vi "KAL Daten loggen.vi"(4 "Aktionen MFC loggen":T1, 6 "TimeOUT":bool, 7 "Komponente":string, 8 "Kalibrieren Erfolgreich":bool, 9 "Prüfgaskonzentration":sgl, 10 "Kalibrierwert":sgl, 11 "Rohwert":sgl) -> (3 "Pfad+Name":path)   [LabVIEW 2020, in "Auto Kalibrieren.lvlib"]
uses:
  Auto Kalibrieren.lvlib
  KAL Daten loggen Aktionen.ctl
  Allgemein/allgemeine Sub-VIs.lvlib
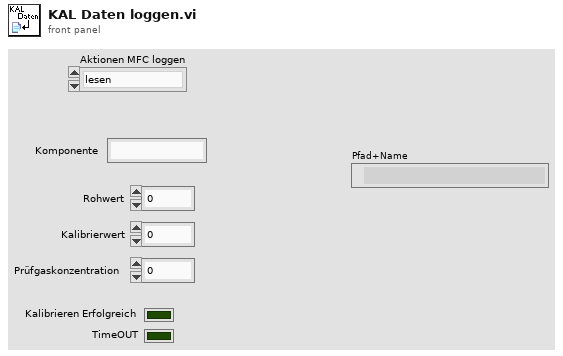
[diagram p1: front panel]
types:
  T1 = typedef "Auto Kalibrieren.lvlib/KAL Daten loggen Aktionen.ctl" = enum16{"lesen", "initialisieren", "loggen"}
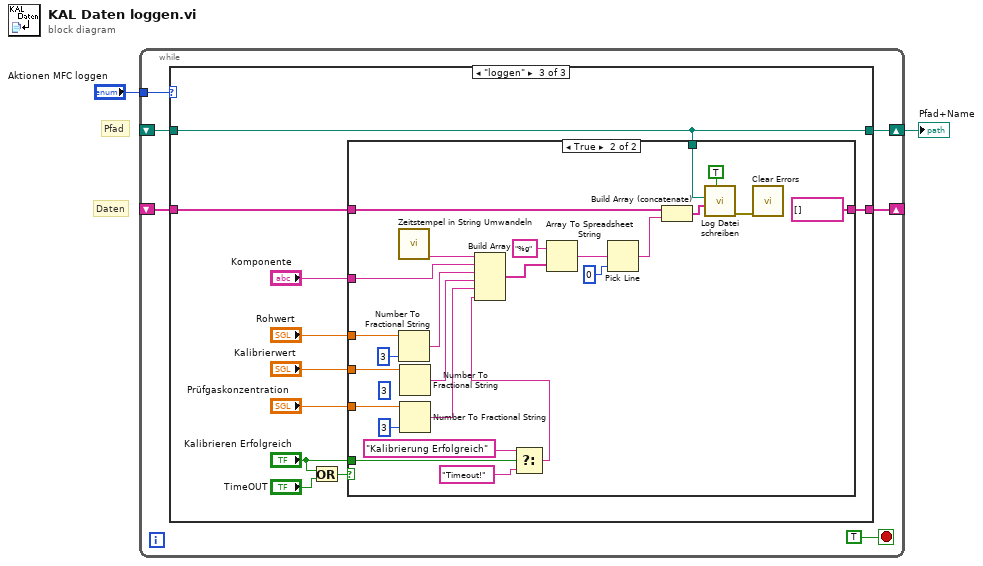
[diagram p0: block diagram]
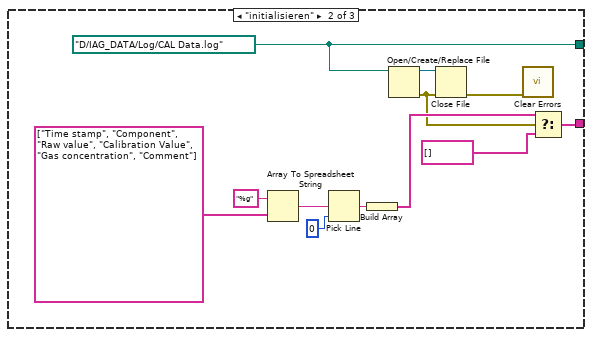
[diagram p3: hidden frame]
diagram:
  # "Pfad"
  # "Daten"
  n1 = while {
    tunnel: "Aktionen MFC loggen" -> [w7]
    shift-right: [w5] -> w1
    shift-left: _ -> [w6]
    shift-right: [w4] -> _
    shift-left: _ -> [w3]
    stop <- TRUE stop-if-true
    n2 = case shown="\"loggen\"" w7 {
      tunnel: w6 -> [w10 _ w32]
      tunnel: [w10 w11 w32] -> w5
      tunnel: [w9 w15 w31] -> w4
      tunnel: w3 -> [w9 _ w30]
      frame "lesen", Default {
      }
      frame "initialisieren" {
        w11 = path "D:/IAG_DATA/Log/CAL Data.log" ("Pfad+Name")
        n3 = Array To Spreadsheet String(array=string[] ["Time stamp", "Component", "Raw value", "Calibration Value", "Gas concentration", "Comment"], 3:"%g" ("Format-String")) -> (spreadsheet string=w20:string)  [unwired: 1 in]
        n4 = Pick Line(multi-line string=w20, line index=0 ("Zeilenindex")) -> (output string=w18:string)  [unwired: 1 in]
        n5 = Build Array(w18) -> (w16:string[])
        n6 = Open/Create/Replace File(file path (use dialog)=w11) -> (refnum out=w13:refnum<file>, error out=w12:errorcluster)  [unwired: 5 in, 1 out]
        n7 = Close File(refnum=w13, error in=w12) -> (error out=w17:errorcluster)  [unwired: 1 out]
        n8 = call <vilib>:"Clear Errors.vi"("error in (no error)"=w17) -> ()  [unwired: 5 in, 2 out]
        n9 = Select(t=w16, s=w12, f=string[] [] ("Angehängtes Array")) -> (s? t:f=w15:string[])
      }
      frame "loggen" {
        n10 = Or(x="Kalibrieren Erfolgreich", y="TimeOUT") -> (x .or. y?=w24:bool)
        n11 = case shown="True" w24 {
          tunnel: w32 -> [_ w58]
          tunnel: [w33 string[] []] -> w31
          tunnel: w30 -> [w33 w56]
          tunnel: "Rohwert" -> [_ w48]
          tunnel: "Kalibrierwert" -> [_ w46]
          tunnel: "Prüfgaskonzentration" -> [_ w44]
          tunnel: "Komponente" -> [_ w43]
          tunnel: "Kalibrieren Erfolgreich" -> [_ w39]
          frame False {
          }
          frame True {
            (unwired) i16 3 ("Genauigkeit (6)")
            n12 = call "Zeitstempel in String Umwandeln.vi"() -> ("Zeitstempel"=w55:string)  [unwired: 10 in, 1 out]
            n13 = Number To Fractional String(number=w48, precision (6)=i16 3 ("Genauigkeit (6)")) -> (F-format string=w42:string)  [unwired: 2 in]
            n14 = Number To Fractional String(number=w46) -> (F-format string=w41:string)  [unwired: 3 in]
            n15 = Number To Fractional String(number=w44, precision (6)=i16 3 ("Genauigkeit (6)")) -> (F-format string=w40:string)  [unwired: 2 in]
            n16 = Select(t="Kalibrierung Erfolgreich", s=w39, f="Timeout!") -> (s? t:f=w36:string)
            n17 = Build Array(w55, w43, w42, w41, w40, w36) -> (w51:string[])
            n18 = Array To Spreadsheet String(array=w51, 3:"%g" ("Format-String")) -> (spreadsheet string=w53:string)  [unwired: 1 in]
            n19 = Pick Line(multi-line string=w53, line index=0 ("Zeilenindex")) -> (output string=w49:string)  [unwired: 1 in]
            n20 = Build Array (concatenate)(w56, w49) -> (w35:string[])
            n21 = call "Log Datei schreiben.vi"("An Datei Anhängen?"=TRUE, "Array"=w35, "Dateipfad"=w58) -> ("error out"=w34:errorcluster)  [unwired: 8 in]
            n22 = call <vilib>:"Clear Errors.vi"("error in (no error)"=w34) -> ()  [unwired: 5 in, 2 out]
          }
        }
      }
    }
  }
  "Pfad+Name" <- w1
